vi "personalities.vi"(9 "Personality":T2, 10 "Lifetime":i64) -> (1 "move":i32, 2 "threats":T1[](array[typedef]), 3 "no threats":T1[](array[typedef]))   [LabVIEW 2017]
uses:
  Common/personality.ctl
  Type Defs/Action Enum.ctl
  Type Defs/SB Type Defs.lvlib
  Common/JFD_Common.lvlib
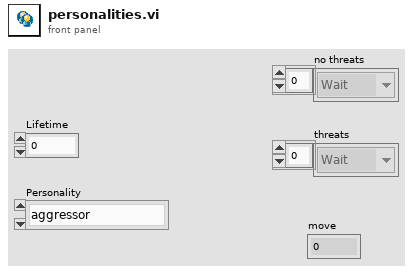
[diagram p1: front panel]
types:
  T1 = typedef "SB Type Defs.lvlib/Action Enum.ctl" = enum16{"Wait", "Move", "Attack", "Replicate"}
  T2 = typedef "JFD_Common.lvlib/personality.ctl" = enum16{"aggressor", "replicator"}
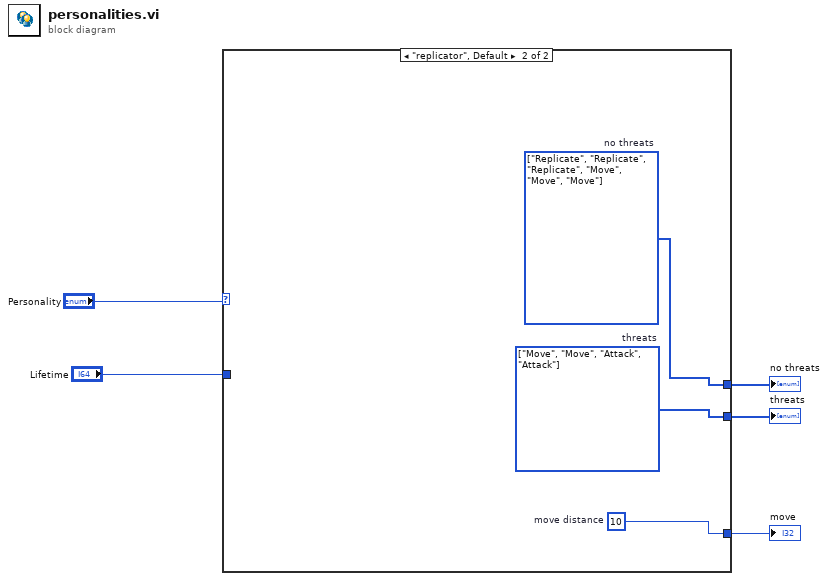
[diagram p0: block diagram]
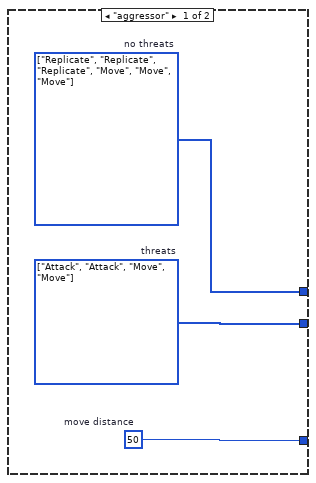
[diagram p2: hidden frame]
diagram:
  n1 = case shown="\"replicator\", Default" "Personality" {
    tunnel: [w8 w11] -> w2
    tunnel: [w7 w10] -> w3
    tunnel: [w6 w9] -> w4
    tunnel: "Lifetime" -> [_ _]
    frame "aggressor" {
      w6 = 50  # move distance
      w7 = T1[] [enum."Attack", enum."Attack", enum."Move", enum."Move"] items=["Wait", "Move", "Attack", "Replicate"]  # threats
      w8 = T1[] [enum."Replicate", enum."Replicate", enum."Replicate", enum."Move", enum."Move", enum."Move"] items=["Wait", "Move", "Attack", "Replicate"]  # no threats
    }
    frame "replicator", Default {
      w9 = 10  # move distance
      w10 = T1[] [enum."Move", enum."Move", enum."Attack", enum."Attack"] items=["Wait", "Move", "Attack", "Replicate"]  # threats
      w11 = T1[] [enum."Replicate", enum."Replicate", enum."Replicate", enum."Move", enum."Move", enum."Move"] items=["Wait", "Move", "Attack", "Replicate"]  # no threats
    }
  }
  "move" <- w4
  "threats" <- w3
  "no threats" <- w2
